vi "Main  - vision.vi"() -> ()   [LabVIEW 2018]
uses:
  <vilib>/DAQmx/write.llb/DAQmx Write (Counter 1D Frequency NChan 1Samp).vi
  <vilib>/DAQmx/configure/timing.llb/DAQmx Timing (Implicit).vi
  <vilib>/vision/driver/NI_Vision_Acquisition_Software.lvlib
  <vilib>/userDefined/High Color/IMAQdx.ctl
  <vilib>/vision/driver/IMAQdx.llb/IMAQdx Acquisition Mode.ctl
  typedef/Parametros control.ctl
  typedef/Selector control.ctl
panel:
  out "Tiempo de ciclo":u32
  out "Image":T1(plugin-control)
  out "Respuesta":cluster{"[0]":dbl, "[1]":dbl, "[2]":dbl}(graph)
  in  "Tipo de control":T2=enum."On-off hist."
  in  "Parametros":T3={"Setpoint"=0.0, "Variable de proceso"=0.0, "Frecuencia PWM"=50.0, "Ciclo de trabajo PWM"=0.5000025, "V. histeresis (grados)"=0.0, "Ganacias PID"={"proportional gain (Kc)"=1.0, "integral time (Ti, min)"=inf, "derivative time (Td, min)"=0.0}} {"Variable de proceso" min=2.5e-06 max=1.0 step=0.1; "V. histeresis (grados)" min=2.5e-06 max=1.0 step=0.1}
  in  "Setpoint":dbl(knob) scale=-120.0..120.0
  out "Variable de proceso":dbl(knob) scale=-135.0..135.0
  in  "stop":bool
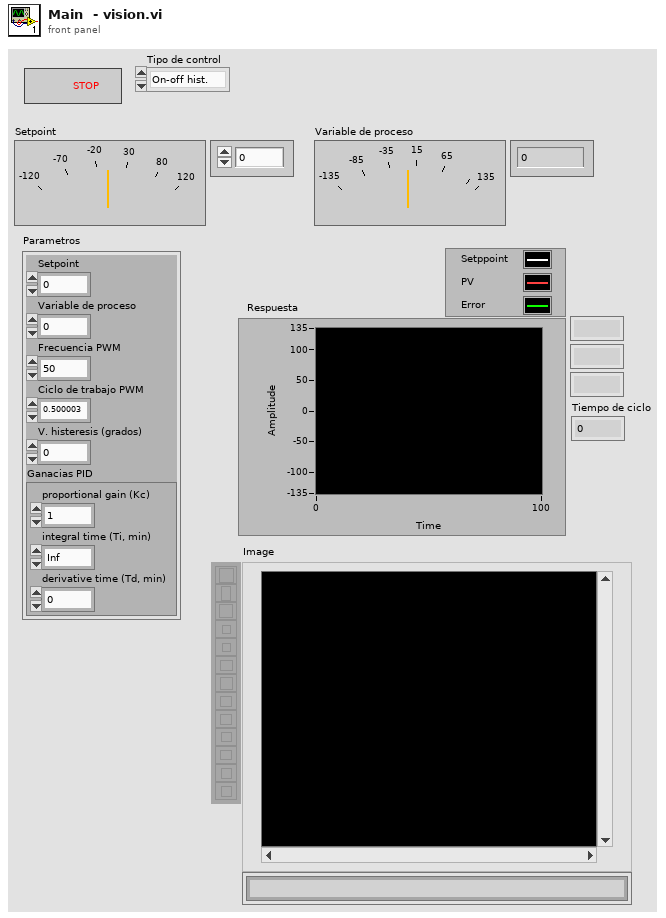
[diagram p1: front panel]
types:
  T1 = typedef "IMAQ Image.ctl" = refnum<image>
  T2 = typedef "Selector control.ctl" = enum16{"On-off", "On-off hist.", "PID"}
  T3 = typedef "Parametros control.ctl" = cluster{"Setpoint":dbl, "Variable de proceso":dbl, "Frecuencia PWM":dbl, "Ciclo de trabajo PWM":dbl, "V. histeresis (grados)":dbl, "Ganacias PID":cluster{"proportional gain (Kc)":dbl, "integral time (Ti, min)":dbl, "derivative time (Td, min)":dbl}}
  T4 = typedef "NI_Vision_Acquisition_Software.lvlib/IMAQdx Acquisition Mode.ctl" = enum32{"One Shot", "Continuous"}
  T5 = typedef "IMAQdx.ctl" = refnum<k21>
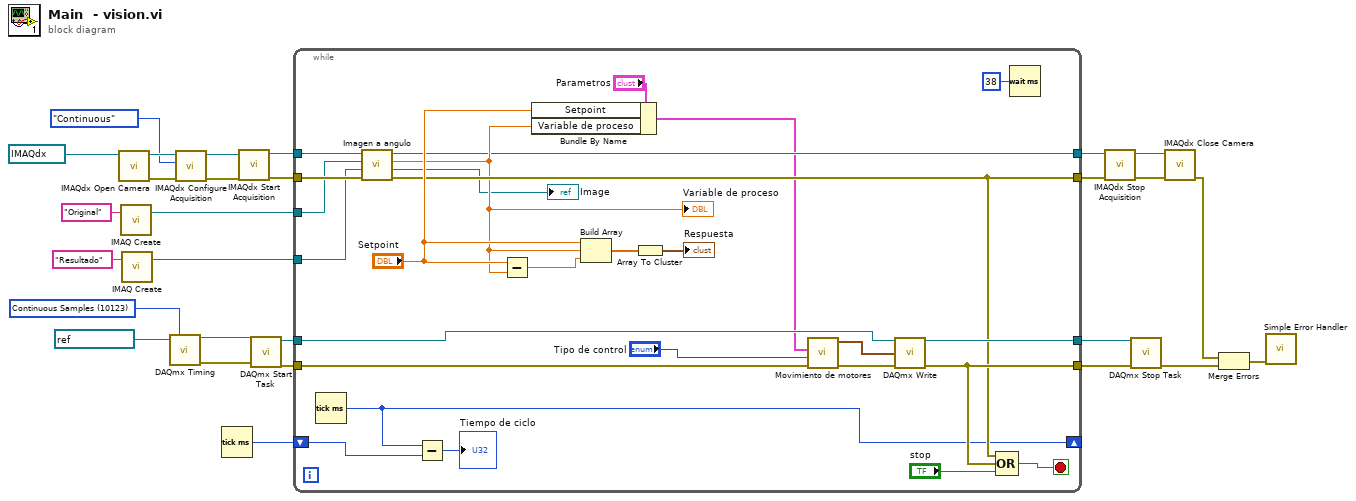
[diagram p0: block diagram]
diagram:
  w23 = 10123 items=["Finite Samples"=10178, "Continuous Samples"=10123, "Hardware Timed Single Point"=12522] ("sample mode")
  n1 = call <vilib>:"IMAQdx Open Camera.vi"("Session In"=T5 "cam0") -> ("error out"=w17:errorcluster, "Session Out"=w16:T5)  [unwired: 9 in]
  n2 = call "IMAQ Create"("Image Name"="Original") -> ("New Image"=w8:T1)  [unwired: 4 in, 1 out]
  n3 = call "IMAQ Create"("Image Name"="Resultado") -> ("New Image"=w7:T1)  [unwired: 4 in, 1 out]
  n4 = call-poly <vilib>:"DAQmx Timing.vi"("task/channels in"=refnum<k21> "CW, CCW" ("DAQmx Global Channel"), "sample mode"=w23) -> ("task out"=w25:refnum<k21>, "error out"=w24:errorcluster)  [unwired: 12 in]
  n5 = call <vilib>:"IMAQdx Configure Acquisition.vi"("error in"=w17, "Continuous?"=IMAQdx_Acquisition_Mode."Continuous", "Session In"=w16) -> ("error out"=w14:errorcluster, "Session Out"=w13:T5)  [unwired: 7 in]
  n6 = Tick Count (ms)() -> (millisecond timer value=w1:u32)
  n7 = call <vilib>:"IMAQdx Start Acquisition.vi"("error in"=w14, "Session In"=w13) -> ("error out"=w9:errorcluster, "Session Out"=w12:T5)  [unwired: 8 in]
  n8 = call <vilib>:"DAQmx Start Task.vi"("task/channels in"=w25, "error in"=w24) -> ("task out"=w28:refnum<k21>, "error out"=w27:errorcluster)  [unwired: 12 in]
  n9 = while {
    tunnel: [w40] -> w6
    tunnel: w28 -> [w52]
    tunnel: w27 -> [w53]
    tunnel: [w49] -> w22
    tunnel: [w48] -> w21
    tunnel: w12 -> [w38]
    tunnel: w9 -> [w37]
    tunnel: w8 -> [w34]
    tunnel: w7 -> [w36]
    tunnel: [w35] -> w4
    shift-right: [w31] -> _
    shift-left: w1 -> [w32]
    stop <- w50 stop-if-true
    n10 = Tick Count (ms)() -> (millisecond timer value=w31:u32)
    n11 = call "Imagen a angulo.vi"("error in (no error)"=w37, "Imagen destino (in)"=w36, "Imagen original"=w34, "Sesion de camara (in)"=w38) -> ("error out"=w40:errorcluster, "Imagen destino (out)"=→"Image":T1, "Variable de proceso"=w39:dbl, "Sesion de camara (out)"=w35:T5)  [unwired: 4 in]
    "Variable de proceso" <- w39
    n12 = Subtract(x=w31, y=w32) -> (x-y=→"Tiempo de ciclo":u32)
    n13 = Subtract(x="Setpoint", y=w39) -> (x-y=w44:dbl)
    n14 = Bundle By Name(cluster="Parametros", "Setpoint"="Setpoint", "Variable de proceso"=w39) -> (w29:T3)
    n15 = Build Array("Setpoint", w39, w44) -> (w46:dbl[])
    n16 = Array To Cluster(array=w46) -> (cluster=→"Respuesta":cluster{"[0]":dbl, "[1]":dbl, "[2]":dbl})
    n17 = call "Movimiento de motores.vi"("Tipo de control"="Tipo de control", "Parametros de control"=w29) -> ("Salida a motores"=w51:cluster{"duty cycle":dbl, "frequency":dbl}[])  [unwired: 8 in, 1 out]
    n18 = call-poly <vilib>:"DAQmx Write.vi"("task/channels in"=w52, "data"=w51, "error in"=w53) -> ("task out"=w48:refnum<k21>, "error out"=w49:errorcluster)  [unwired: 10 in, 1 out]
    n19 = Compound Arithmetic op=OR(w40, w49, "stop") -> (w50:bool)
    n20 = Wait (ms)(milliseconds to wait=u32 38) -> ()  [unwired: 1 out]
  }
  n21 = call <vilib>:"IMAQdx Stop Acquisition.vi"("error in"=w6, "Session In"=w4) -> ("error out"=w5:errorcluster, "Session Out"=w3:T5)  [unwired: 8 in]
  n22 = call <vilib>:"DAQmx Stop Task.vi"("task/channels in"=w21, "error in"=w22) -> ("error out"=w20:errorcluster)  [unwired: 12 in, 1 out]
  n23 = call <vilib>:"IMAQdx Close Camera.vi"("error in"=w5, "Session In"=w3) -> ("error out"=w2:errorcluster)  [unwired: 9 in]
  n24 = Merge Errors(w2, w20) -> (w19:errorcluster)
  n25 = call <vilib>:"Simple Error Handler.vi"("error in (no error)"=w19) -> ()  [unwired: 4 in, 5 out]
